vi "GenerateData.vi"(8 "error in (no error)":errorcluster, 11 "Numeric in":refnum<class "Numeric.lvclass">) -> (0 "error out":errorcluster, 3 "Numeric out":refnum<class "Numeric.lvclass">)   [LabVIEW 2023, in "Numeric.lvclass"]
uses:
  Numeric.lvclass
  <vilib>/numeric/Random Number (Range) DBL.vi
  Numeric.lvclass/Numeric.ctl
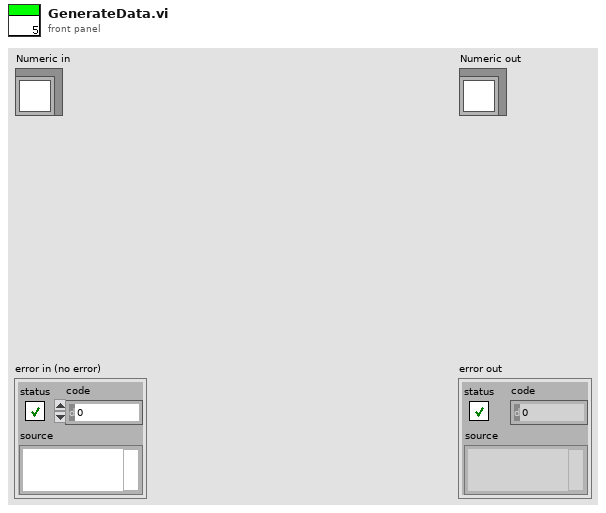
[diagram p1: front panel]
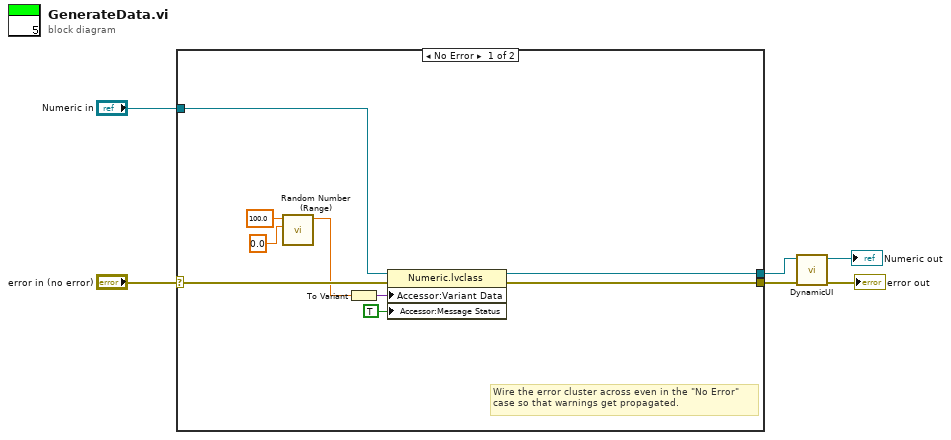
[diagram p0: block diagram]
diagram:
  n1 = case shown="No Error" "error in (no error)" {
    selector: "error in (no error)" -> [w15 w17]
    tunnel: [w7 w17] -> w4
    tunnel: [w8 w16] -> w2
    tunnel: "Numeric in" -> [w10 w16]
    frame No Error {
      # "Wire the error cluster across even in the \"No Error\"\ncase so that warnings get propagated."
      n2 = call-poly <vilib>:"Random Number (Range).vi"("lower bound (0)"=0.0, "upper bound (100)"=100.0) -> ("number"=w12:dbl)  [unwired: 9 in]
      n3 = To Variant(anything=w12) -> (Variant=w11:variant)
      n4 = property class="Numeric.lvclass"(reference=w10, error in=w15, "Accessor:Variant Data"=w11, "Accessor:Message Status"=TRUE ("Message Status")) -> (reference out=w8:refnum<class "Numeric.lvclass">, error out=w7:errorcluster)
    }
    frame Error {
    }
  }
  n5 = call "DynamicUI.vi"("error in (no error)"=w4, "Numeric in"=w2) -> ("error out"=→"error out":errorcluster, "Numeric out"=→"Numeric out":refnum<class "Numeric.lvclass">)  [unwired: 8 in]
